vi "TalonData.vi"(9 "Output Speed":dbl, 10 "Seconds":dbl) -> (0 "Total":dbl[](array[numeric]), 1 "Average Signed Error":dbl[](array[numeric]), 2 "Max Error":dbl[](array[numeric]), 3 "Average Error":dbl[](array[numeric]))   [LabVIEW 2016]
uses:
  Robot Global Data.vi
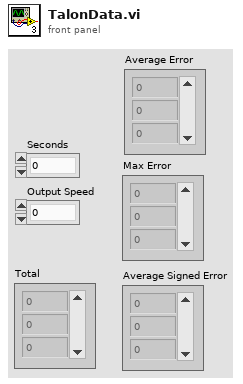
[diagram p1: front panel]
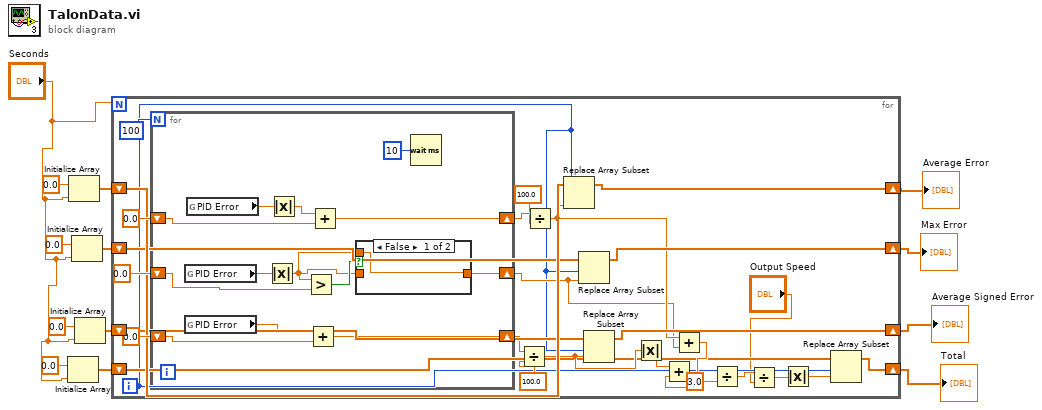
[diagram p0: block diagram]
diagram:
  n1 = Initialize Array(0.0 ("element"), "Seconds") -> (w6:dbl[])
  n2 = Initialize Array(0.0 ("element"), "Seconds") -> (w13:dbl[])
  n3 = Initialize Array(0.0 ("element"), "Seconds") -> (w9:dbl[])
  n4 = Initialize Array(0.0 ("element"), "Seconds") -> (w8:dbl[])
  n5 = for {
    N: "Seconds" -> [_]
    shift-right: [w36] -> w5
    shift-left: w13 -> [w37]
    shift-right: [w35] -> w3
    shift-left: w9 -> [w32]
    shift-right: [w34] -> w2
    shift-left: w8 -> [w33]
    shift-right: [w20] -> w4
    shift-left: w6 -> [w22]
    i -> [w21]
    n6 = for {
      N: 100 -> [_]
      shift-right: [w51] -> w31
      shift-left: 0.0 -> [w52]
      shift-right: [w48] -> w25
      shift-left: 0.0 -> [w50]
      shift-right: [w47] -> w29
      shift-left: 0.0 -> [w46]
      n7 = global read "Robot Global Data.vi" "PID Error"() -> (w43:dbl)
      n8 = global read "Robot Global Data.vi" "PID Error"() -> (w45:dbl)
      n9 = global read "Robot Global Data.vi" "PID Error"() -> (w54:dbl)
      n10 = Absolute Value(x=w43) -> (abs(x)=w42:dbl)
      n11 = Absolute Value(x=w54) -> (abs(x)=w53:dbl)
      n12 = Greater?(x=w42, y=w50) -> (0:w49:bool)
      n13 = Add(x=w45, y=w46) -> (x+y=w47:dbl)
      n14 = Add(x=w53, y=w52) -> (x+y=w51:dbl)
      n15 = case shown="False" w49 {
        tunnel: w42 -> [_ w56]
        tunnel: [w55 w56] -> w48
        tunnel: w42 -> [w55 _]
        frame False {
        }
        frame True {
        }
      }
      n16 = Wait (ms)(milliseconds to wait=u32 10) -> ()  [unwired: 1 out]
    }
    n17 = Divide(x=w29, y=100.0) -> (x/y=w27:dbl)
    n18 = Divide(x=w31, y=100.0 ("x")) -> (x/y=w26:dbl)
    n19 = Replace Array Subset(array=w37, new element=w26, index=w21) -> (w36:dbl[])
    n20 = Replace Array Subset(array=w32, new element=w25, index=w21) -> (w35:dbl[])
    n21 = Replace Array Subset(array=w33, new element=w27, index=w21) -> (w34:dbl[])
    n22 = Absolute Value(x=w27) -> (abs(x)=w24:dbl)
    n23 = Add(x=w26, y=w25) -> (x+y=w23:dbl)
    n24 = Add(x=w24, y=w23) -> (x+y=w19:dbl)
    n25 = Divide(x=w19, y=3.0) -> (x/y=w17:dbl)
    n26 = Divide(x=w17, y="Output Speed") -> (x/y=w16:dbl)
    n27 = Absolute Value(x=w16) -> (abs(x)=w15:dbl)
    n28 = Replace Array Subset(array=w22, new element=w15, index=w21) -> (w20:dbl[])
  }
  "Average Error" <- w5
  "Total" <- w4
  "Max Error" <- w3
  "Average Signed Error" <- w2
